vi "DEMO2_lvlibp.vi"() -> ()   [LabVIEW 2022 SP3]
panel:
  out "error out":errorcluster
  # "#调用打包库"
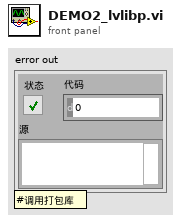
[diagram p1: front panel]
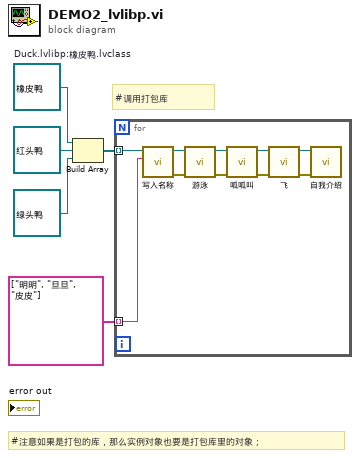
[diagram p0: block diagram]
diagram:
  w3 = refnum<class "橡皮鸭.lvclass"> refnum  # Duck.lvlibp:橡皮鸭.lvclass
  # "#调用打包库"
  # "#注意如果是打包的库，那么实例对象也要是打包库里的对象；"
  n1 = Build Array(w3, refnum<class "红头鸭.lvclass"> refnum ("Duck.lvlibp:红头鸭.lvclass"), refnum<class "绿头鸭.lvclass"> refnum ("Duck.lvlibp:绿头鸭.lvclass")) -> (w4:refnum<class "鸭子.lvclass">[])
  n2 = for {
    tunnel: string[] ["明明", "旦旦", "皮皮"] -> [w7] mode=indexing
    tunnel: w4 -> [w6] mode=indexing
    n3 = call "写入名称.vi"("名称"=w7, "鸭子输入"=w6) -> ("error out"=w14:errorcluster, "鸭子输出"=w15:refnum<class "鸭子.lvclass">)  [unwired: 8 in]
    n4 = call-dynamic "游泳.vi"("error in (no error)"=w14, "鸭子 输入"=w15) -> ("error out"=w12:errorcluster, "鸭子 输出"=w13:refnum<class "鸭子.lvclass">)  [unwired: 8 in]
    n5 = call-dynamic "呱呱叫.vi"("error in (no error)"=w12, "鸭子 输入"=w13) -> ("error out"=w10:errorcluster, "鸭子 输出"=w11:refnum<class "鸭子.lvclass">)  [unwired: 8 in]
    n6 = call-dynamic "飞.vi"("error in (no error)"=w10, "鸭子 输入"=w11) -> ("error out"=w8:errorcluster, "鸭子 输出"=w9:refnum<class "鸭子.lvclass">)  [unwired: 8 in]
    n7 = call-dynamic "自我介绍.vi"("error in (no error)"=w8, "鸭子 输入"=w9) -> ()  [unwired: 8 in, 2 out]
  }
